vi "Actor Core.vi"(8 "error in":errorcluster, 11 "Elevator Controller Actor in":refnum<class "Sim Display Console Actor.lvclass">) -> (0 "error out":errorcluster, 3 "Actor out":refnum<class "Actor.lvclass">)   [LabVIEW 2022 SP3, in "Sim Display Console Actor.lvlib" / "Sim Display Console Actor.lvclass"]
doc: "(<B>Filename</B>: Actor Framework.lvlib:Actor.lvclass:Actor Core.vi)\n\nReceives messages to the actor, reacts to them, and initiates any error handling that may shut the actor down.\n\nDescendant classes may override this VI to append parallel tasks for the actor to complete while it handles messages. Overrides use the Call Parent Class Method node."
uses:
  Sim Display Console Actor.lvclass
  C:/Program Files/National Instruments/LabVIEW 2022/vi.lib/ActorFramework/Actor/Actor.lvclass
  <vilib>/ActorFramework/Actor/Actor.lvclass
  Floor -Enum.ctl
  Elevator Direction.ctl
  Sim Display Console Actor.lvclass/Sim Display Console Actor.ctl
  <vilib>/ActorFramework/Actor/Actor.lvclass/Actor.ctl
  <vilib>/ActorFramework/Message Enqueuer/Message Enqueuer.lvclass/Message Enqueuer.ctl
  <vilib>/ActorFramework/Message Enqueuer/Init from Existing Queue.vi
  <vilib>/ActorFramework/Message Enqueuer/Enqueue.vi
  <vilib>/ActorFramework/Stop Msg/Stop Msg.lvclass
  C:/Program Files/National Instruments/LabVIEW 2022/vi.lib/ActorFramework/Message/Message.lvclass
  <vilib>/ActorFramework/Message Priority Queue/Priority Enqueue.vi
  Display Console Actor/Display Console Actor/Display Console Actor.lvclass
  <vilib>/ActorFramework/Message Enqueuer/Message Enqueuer.lvclass
panel:
  out "Emergency":bool
  out "Elevator Direction":T1
  out "Door Open":bool
  out "Elevator Location":T2
  out "Timing":dbl
  # "[Covers: UI3] \n[Covers: UI3A] \n[Covers: UI3A1] \n[Covers: UI3A2] \n[Covers: UI3B] \n[Covers: UI3C] \n[Covers: UI3D] \n[Covers: UI3D1] \n[Covers: UI3D2] \n[Covers: UI3E]"
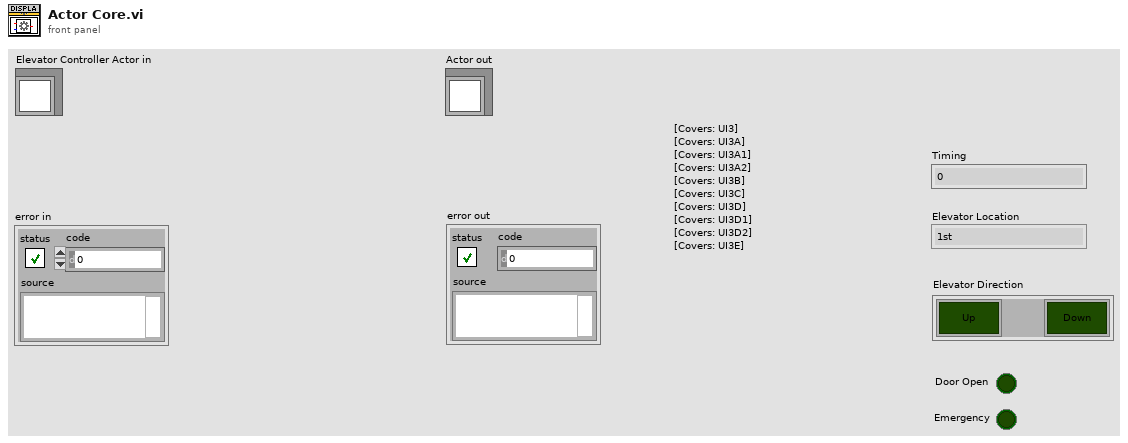
[diagram p1: front panel]
types:
  T1 = typedef "Sim Display Console Actor.lvlib/Sim Display Console Actor.lvclass/Elevator Direction.ctl" = cluster{"Up":bool, "Down":bool}
  T2 = typedef "Sim Display Console Actor.lvlib/Sim Display Console Actor.lvclass/Floor -Enum.ctl" = enum16{"1st", "2nd", "3rd", "4th"}
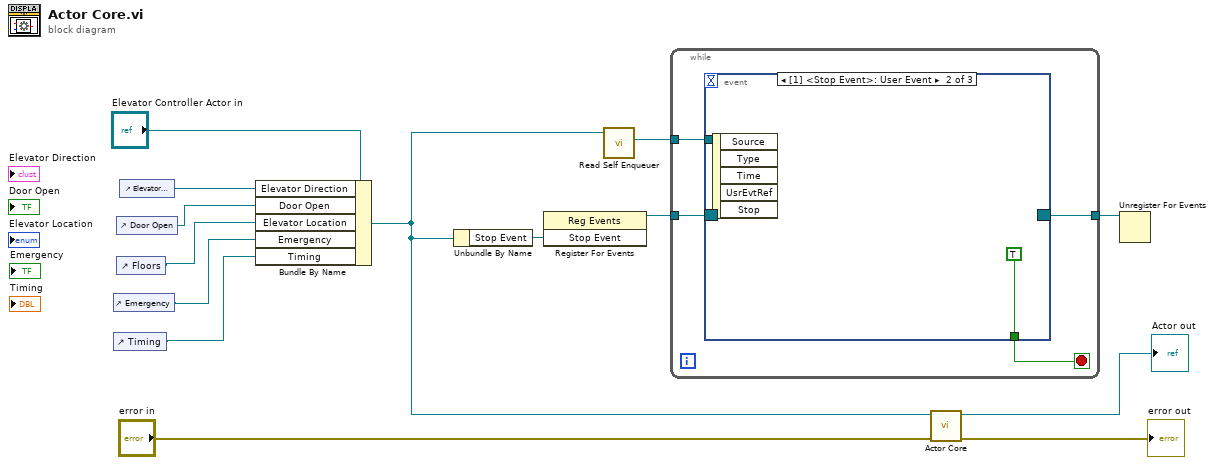
[diagram p0: block diagram]
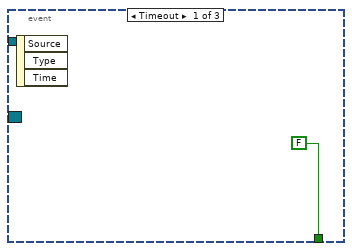
[diagram p2: hidden frame]
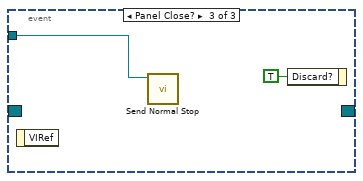
[diagram p3: hidden frame]
diagram:
  n1 = control-ref of="Emergency"() -> (w2:refnum<vi>)
  n2 = control-ref of="Timing"() -> (w1:refnum<vi>)
  n3 = control-ref of="Door Open"() -> (w4:refnum<vi>)
  n4 = control-ref of="Floors"() -> (w3:refnum<vi>)
  n5 = control-ref of="Elevator Direction"() -> (w6:refnum<vi>)
  n6 = Bundle By Name(cluster="Elevator Controller Actor in", "Elevator Direction"=w6, "Door Open"=w4, "Elevator Location"=w3, "Emergency"=w2, "Timing"=w1) -> (w5:refnum<class "Sim Display Console Actor.lvclass">)
  n7 = Unbundle By Name(w5) -> ("Stop Event"=w11:refnum<user-event>)
  n8 = register-events(w11) -> (reference out=w10:refnum<event-registration>)  [unwired: 2 in, 1 out]
  n9 = call <vilib>:"Read Self Enqueuer.vi"("Actor"=w5) -> ("Self Enqueuer"=w8:refnum<class "Message Enqueuer.lvclass">)  [unwired: 10 in]
  n10 = while {
    tunnel: w10 -> [w17]
    tunnel: [w16] -> w9
    tunnel: w8 -> [w15]
    stop <- w18 stop-if-true
    n11 = event shown="[1] <Stop Event>: User Event" {
      selector: w17 -> [_ _ _]
      dyn-events: [_ _ _] -> w16
      timeout: _ -> [_ _ _]
      tunnel: [FALSE TRUE _] -> w18
      tunnel: w15 -> [_ _ w21]
      event Timeout {
        n12 = event-data() -> ()  [unwired: 1 in, 3 out]
      }
      event User Event {
        n13 = event-data() -> ()  [unwired: 1 in, 5 out]
      }
      event Panel Close? {
        n14 = event-data() -> ()  [unwired: 1 in, 1 out]
        n15 = call <vilib>:"Send Normal Stop.vi"("Message Enqueuer"=w21) -> ()  [unwired: 10 in, 1 out]
        n16 = event-data("Discard?"=TRUE) -> ()  [unwired: 1 in, 1 out]
      }
    }
  }
  n17 = call-parent "Actor Core.vi"("error in"="error in", "Actor in"=w5) -> ("error out"=→"error out":errorcluster, "Actor out"=→"Actor out":refnum<class "Actor.lvclass">)  [unwired: 8 in]
  n18 = Unregister For Events(event registration refnum=w9) -> ()  [unwired: 1 in, 1 out]
